vi "Reset Instruments.vi"(8 "error in":errorcluster, 11 "Base Software in":refnum<class "Base Software.lvclass">) -> (0 "error out":errorcluster, 3 "Base Software out":refnum<class "Base Software.lvclass">)   [LabVIEW 2019, in "Base Software.lvlib" / "Main.lvlib" / "Base Software.lvclass"]
uses:
  Project/Base Software.lvclass
  <resource>/objmgr/daqmx.rc
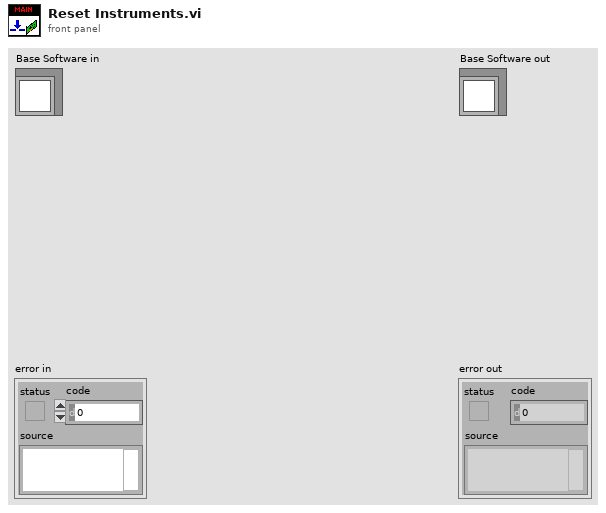
[diagram p1: front panel]
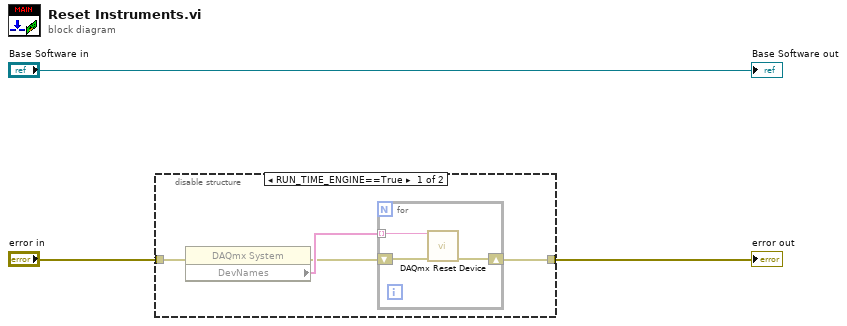
[diagram p0: block diagram]
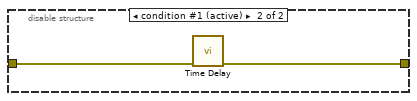
[diagram p2: hidden frame]
diagram:
  n1 = disable-structure shown="RUN_TIME_ENGINE==True" {
    disable-tunnel: "error in" -> [w7 w12]
    disable-tunnel: [w6 w11] -> w2
    frame condition #0 {
      n2 = property class="DAQmx System"(error in=w7) -> (error out=w4:errorcluster, "DevNames"=w5:tag[])  [unwired: 1 in, 1 out]
      n3 = for {
        tunnel: w5 -> [w9] mode=indexing
        shift-right: [w8] -> w6
        shift-left: w4 -> [w10]
        n4 = call <vilib>:"DAQmx Reset Device.vi"("device in"=w9, "error in"=w10) -> ("error out"=w8:errorcluster)  [unwired: 13 in]
      }
    }
    frame condition #1 (active) {
      n5 = call "Time Delay"("error in (no error)"=w12) -> ("error out"=w11:errorcluster)  [unwired: 10 in]
    }
  }
  "error out" <- w2
  "Base Software out" <- "Base Software in"
